vi "generate channel data type tests.vi"(8 "error in (no error)":errorcluster, 11 "Tdms File":refnum<k34>) -> (0 "error out":errorcluster, 3 "Tdms File Out":refnum<k34>)   [LabVIEW 2020]
doc: "Writes alternating segments of 2 sets of channels in the same group. ch1-3 at 1000 per write and 4-6 at 500 per write.\n\nEach pair of writes is alternated between interleaved and decimated data."
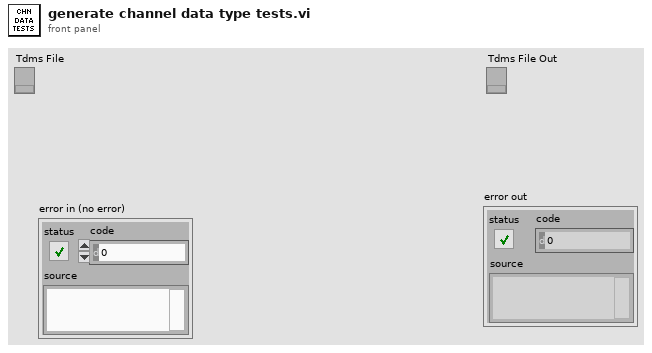
[diagram p1: front panel]
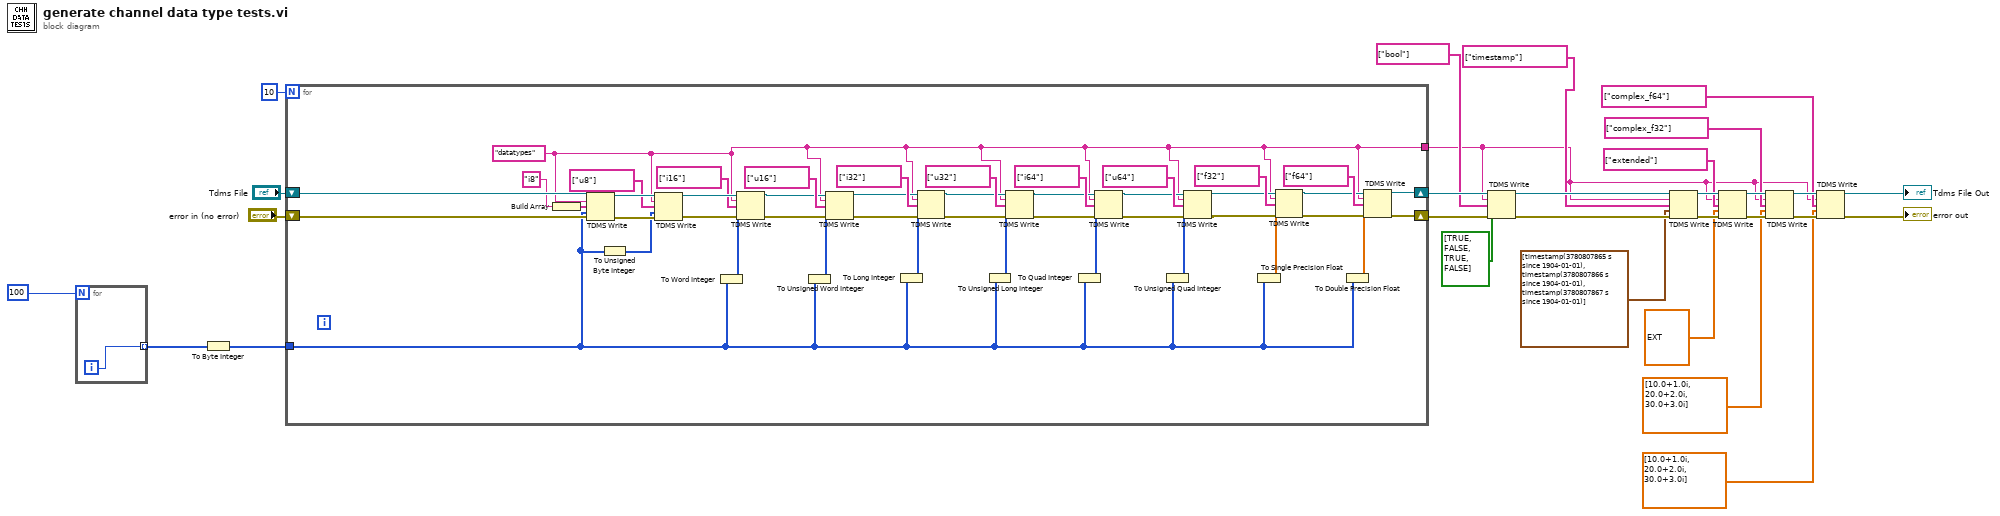
[diagram p0: block diagram]
diagram:
  n1 = for {
    N: 100 ("x") -> [_]
    tunnel: [w30] -> w29 mode=indexing
    i -> [w30]
  }
  n2 = To Byte Integer(number=w29) -> (8bit integer=w27:i8[])
  n3 = for {
    N: 10 -> [_]
    tunnel: w27 -> [w40]
    shift-right: [w42] -> w21
    shift-left: "Tdms File" -> [w74]
    shift-right: [w41] -> w24
    shift-left: "error in (no error)" -> [w71]
    tunnel: [w31] -> w4
    w31 = "datatypes" ("group name in (Untitled)")
    n4 = Build Array("i8") -> (w69:string[])
    n5 = TDMS Write(0:w74, 5:w31, 7:w69, 9:w40, 11:w71) -> (4:w73:refnum<k34>, 15:w72:errorcluster)  [unwired: 1 in, 2 out]
    n6 = To Unsigned Byte Integer(number=w40) -> (unsigned 8bit integer=w67:u8[])
    n7 = TDMS Write(0:w73, 5:w31, 7:string[] ["u8"], 9:w67, 11:w72) -> (4:w66:refnum<k34>, 15:w65:errorcluster)  [unwired: 1 in, 2 out]
    n8 = To Word Integer(number=w40) -> (16bit integer=w39:i16[])
    n9 = TDMS Write(0:w66, 5:w31, 7:string[] ["i16"], 9:w39, 11:w65) -> (4:w62:refnum<k34>, 15:w61:errorcluster)  [unwired: 1 in, 2 out]
    n10 = To Unsigned Word Integer(number=w40) -> (unsigned 16bit integer=w38:u16[])
    n11 = TDMS Write(0:w62, 5:w31, 7:string[] ["u16"], 9:w38, 11:w61) -> (4:w59:refnum<k34>, 15:w58:errorcluster)  [unwired: 1 in, 2 out]
    n12 = To Long Integer(number=w40) -> (32bit integer=w37:i32[])
    n13 = TDMS Write(0:w59, 5:w31, 7:string[] ["i32"], 9:w37, 11:w58) -> (4:w56:refnum<k34>, 15:w55:errorcluster)  [unwired: 1 in, 2 out]
    n14 = To Unsigned Long Integer(number=w40) -> (unsigned 32bit integer=w36:u32[])
    n15 = TDMS Write(0:w56, 5:w31, 7:string[] ["u32"], 9:w36, 11:w55) -> (4:w44:refnum<k34>, 15:w43:errorcluster)  [unwired: 1 in, 2 out]
    n16 = To Quad Integer(1:w40) -> (0:w35:i64[])
    n17 = TDMS Write(0:w44, 5:w31, 7:string[] ["i64"], 9:w35, 11:w43) -> (4:w52:refnum<k34>, 15:w51:errorcluster)  [unwired: 1 in, 2 out]
    n18 = To Unsigned Quad Integer(1:w40) -> (0:w34:u64[])
    n19 = TDMS Write(0:w52, 5:w31, 7:string[] ["u64"], 9:w34, 11:w51) -> (4:w49:refnum<k34>, 15:w48:errorcluster)  [unwired: 1 in, 2 out]
    n20 = To Single Precision Float(number=w40) -> (single precision float=w33:sgl[])
    n21 = TDMS Write(0:w49, 5:w31, 7:string[] ["f32"], 9:w33, 11:w48) -> (4:w46:refnum<k34>, 15:w45:errorcluster)  [unwired: 1 in, 2 out]
    n22 = To Double Precision Float(number=w40) -> (double precision float=w32:dbl[])
    n23 = TDMS Write(0:w46, 5:w31, 7:string[] ["f64"], 9:w32, 11:w45) -> (4:w42:refnum<k34>, 15:w41:errorcluster)  [unwired: 1 in, 2 out]
  }
  n24 = TDMS Write(0:w21, 5:w4, 7:string[] ["bool"] ("channel name(s) in (Untitled)"), 9:bool[] [TRUE, FALSE, TRUE, FALSE], 11:w24) -> (4:w20:refnum<k34>, 15:w22:errorcluster)  [unwired: 1 in, 2 out]
  n25 = TDMS Write(0:w20, 5:w4, 7:string[] ["timestamp"] ("channel name(s) in (Untitled)"), 9:timestamp[] [timestamp(3780807865 s since 1904-01-01), timestamp(3780807866 s since 1904-01-01), timestamp(3780807867 s since 1904-01-01)], 11:w22) -> (4:w15:refnum<k34>, 15:w11:errorcluster)  [unwired: 1 in, 2 out]
  n26 = TDMS Write(0:w15, 5:w4, 7:string[] ["extended"] ("channel name(s) in (Untitled)"), 9:ext[] [1.0, 2.0, 3.0], 11:w11) -> (4:w14:refnum<k34>, 15:w10:errorcluster)  [unwired: 1 in, 2 out]
  n27 = TDMS Write(0:w14, 5:w4, 7:string[] ["complex_f32"] ("channel name(s) in (Untitled)"), 9:csg[] [10.0+1.0i, 20.0+2.0i, 30.0+3.0i], 11:w10) -> (4:w13:refnum<k34>, 15:w9:errorcluster)  [unwired: 1 in, 2 out]
  n28 = TDMS Write(0:w13, 5:w4, 7:string[] ["complex_f64"] ("channel name(s) in (Untitled)"), 9:cdb[] [10.0+1.0i, 20.0+2.0i, 30.0+3.0i], 11:w9) -> (4:→"Tdms File Out":refnum<k34>, 15:→"error out":errorcluster)  [unwired: 1 in, 2 out]
